vi "Create CORE UI Display Events.vi"(11 "error in":errorcluster) -> (4 "Framework Events":T1, 15 "error out":errorcluster)   [LabVIEW 2015, in "TLB` Template.lvlib"]
doc: "Create resources for UI user events.\n\n<B>Input Parameters</B>\n\n<B>error in</B> describes error conditions that occur before this node runs. This input provides standard error in functionality.\n\n<B>Output Parameters</B>\n\n<B>UI display events out</B> created user events.\n\n<B>error out</B> contains error information. This output provides standard error out functionality."
uses:
  TLB` Template.lvlib
  typedefs/_UI CORE Event References.ctl
  Dependencies/TLB`_Dependencies.lvlib
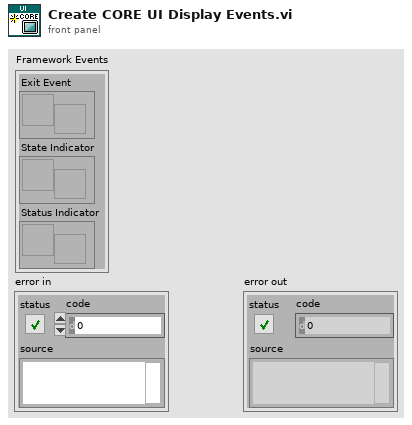
[diagram p1: front panel]
types:
  T1 = typedef "TLB` Template.lvlib/_UI CORE Event References.ctl" = cluster{"Exit Event":refnum<user-event>, "State Indicator":refnum<user-event>, "Status Indicator":refnum<user-event>}
  T2 = typedef "TLB` Template.lvlib/TLB`_Dependencies.lvlib/Exit Event Ref.ctl" = refnum<user-event>
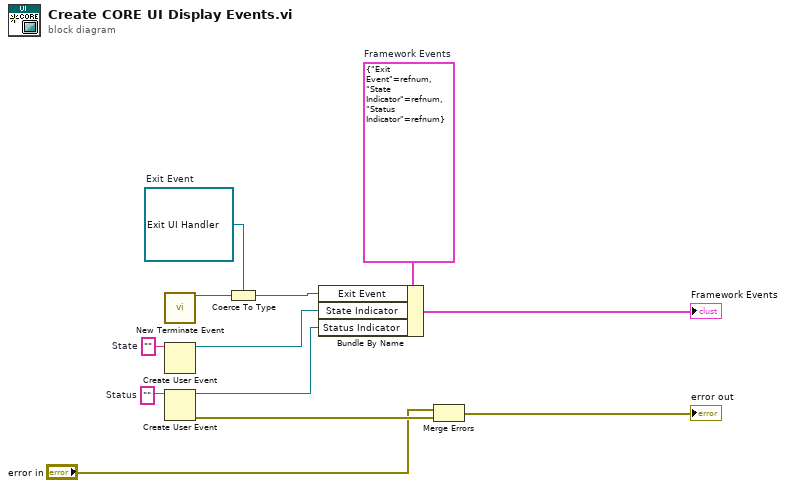
[diagram p0: block diagram]
diagram:
  w1 = refnum<user-event> refnum  # Exit Event
  w9 = ""  # Status
  w11 = T1 {"Exit Event"=refnum, "State Indicator"=refnum, "Status Indicator"=refnum}  # Framework Events
  w12 = ""  # State
  n1 = call "New Terminate Event.vi"() -> ("Exit Event Ref"=w5:T2)  [unwired: 14 in, 1 out]
  n2 = Create User Event(user event datatype=w12) -> (user event=w10:refnum<user-event>)  [unwired: 1 in, 1 out]
  n3 = Create User Event(user event datatype=w9) -> (user event=w7:refnum<user-event>, error out=w8:errorcluster)  [unwired: 1 in]
  n4 = Coerce To Type(0:w5, 1:w1) -> (2:w4:refnum<user-event>)
  n5 = Bundle By Name(cluster=w11, "Exit Event"=w4, "State Indicator"=w10, "Status Indicator"=w7) -> (→"Framework Events":T1)
  n6 = Merge Errors("error in", w8) -> (→"error out":errorcluster)
